vi "AlliGator Create Phasor Plot Additional Data String.vi"(4 "Intensity Weighted ? (F)":bool, 6 "Average Plot Data (F)":bool, 7 "Include Header String (F)":bool, 8 "error in (no error)":errorcluster, 9 "Calibrated Phasor Plot":T2, 10 "Raw Phasor Plot":T4={"Phasor Plot Name"="", "Raw Phasor Plot"=[], "Phasor Frequency"=0.0, "[Decay Metadata]"=[], "Raw Phasor Plot SDV"=[], "Phasor SDV Options"={"Compute Estimated SDV"=FALSE, "# Replicas"=100, "Use Estimated Average Phasor"=FALSE}, "[Calibration Phasor]"=[], "Intensity Array"=[]} {"[Decay Metadata]"."# Folds" min=1; "[Decay Metadata]"."ROI Descriptor"."Contours"."Type" items=["No Selection", "Point", "Line", "Rectangle", "Oval", "Polygon", "Freehand Region", "Annulus", "Unused2", "Unused3", "Broken Line", "Freehand Line", "Rotated Rectangle"]}, 11 "Phasor Plot Exported Data":T1) -> (0 "error out":errorcluster, 3 "Phasor Plot Additional Data String":string)   [LabVIEW 2021, in "AlliGator Phasor Graph.lvlib"]
doc: "Creates a string with all the user-requested phasor plot additional data."
uses:
  AlliGator Phasor Graph.lvlib
  AlliGator Raw Phasor Plot Data v5.ctl
  Phasor/Phasor (g, s).ctl
  AlliGator Decay Metadata v3.ctl
  Decay Analysis/Decay Preprocessing/AlliGator Decay Background Subtraction Info.ctl
  Decay Analysis/Decay Preprocessing/AlliGator Baseline Subtraction Method.ctl
  Graphs/XY Graph/XY Graph Plot Shift Parameters.ctl
  Graphs/XY Graph/XY Graph Plot Shift Method.ctl
  Decay Analysis/Decay Preprocessing/AlliGator Decay Extrapolation Parameters.ctl
  Phasor/Phasor Standard Deviation Options.ctl
  Phasor/Calibration Phasor (m, phi).ctl
  AlliGator Phasor Plot Additional Data List.ctl
  Graphs/XY Graph/XY Graph Plot Data.ctl
  AlliGator Phasor Plot Exported Data Selection.ctl
  d5eb63e0-648c-47d6-be91-64ae69301d4e.vi
  28782bb2-77f9-4fec-b09f-3ba0b8238253.vi
  Strings/Strings.lvlib
  Phasor/Phasor.lvlib
  Phasor Ratio/AlliGator Phasor Ratio.lvlib
  Time/Time.lvlib
  Utilities/Utilities.lvlib
  Math/Math.lvlib
  Decay Analysis/Decay Preprocessing/AlliGator Decay Preprocessing.lvlib
  Graphs/XY Graph/XY Graph Add-Ons.lvlib
panel:
  out "CPU (s)":dbl
  in  "Phasor Plot Exported Data List":T3
  # "see the AlliGator License on the block diagram (Ctrl+E or Window:Show Block Diagram)"
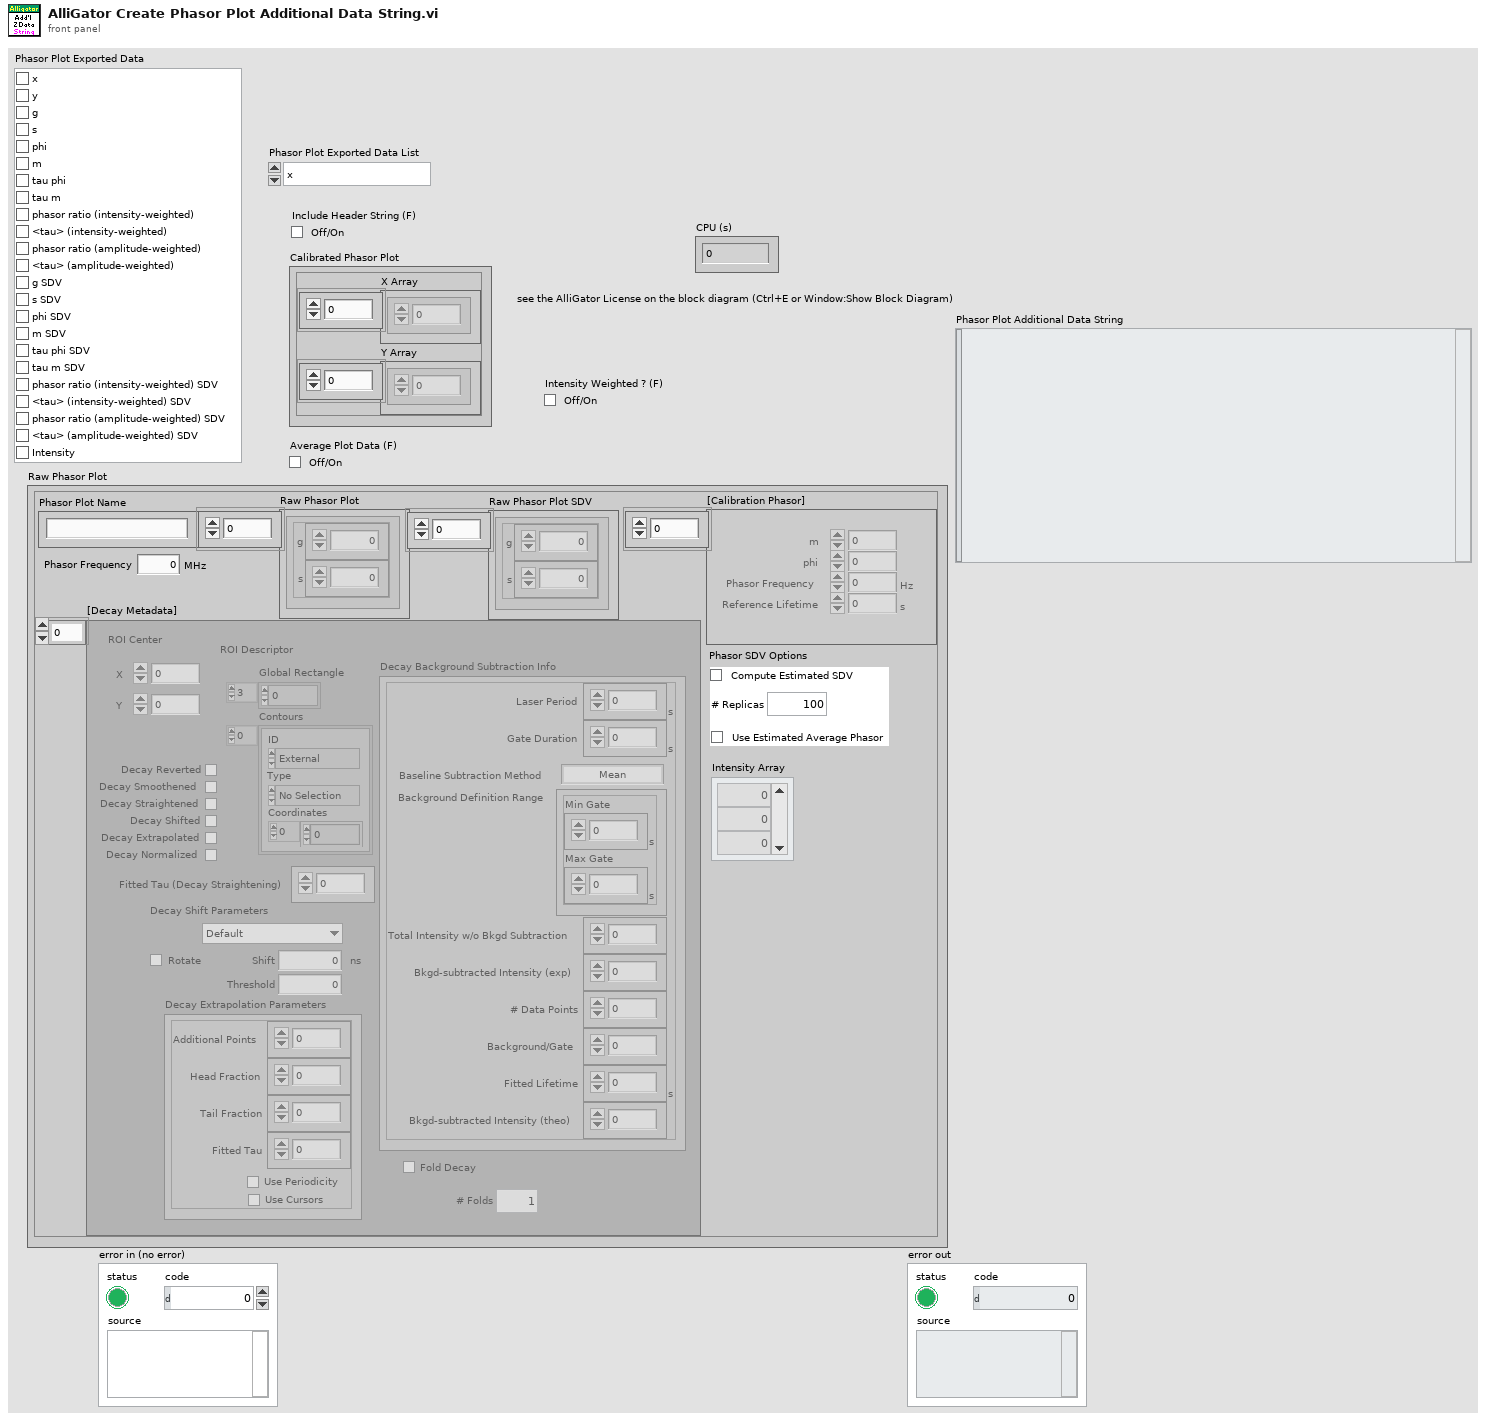
[diagram p1: front panel]
types:
  T1 = typedef "AlliGator Phasor Graph.lvlib/AlliGator Phasor Plot Exported Data Selection.ctl" = cluster{"x":bool, "y":bool, "g":bool, "s":bool, "phi":bool, "m":bool, "tau phi":bool, "tau m":bool, "phasor ratio (intensity-weighted)":bool, "<tau> (intensity-weighted)":bool, "phasor ratio (amplitude-weighted)":bool, "<tau> (amplitude-weighted)":bool, "g SDV":bool, "s SDV":bool, "phi SDV":bool, "m SDV":bool, "tau phi SDV":bool, "tau m SDV":bool, "phasor ratio (intensity-weighted) SDV":bool, "<tau> (intensity-weighted) SDV":bool, "phasor ratio (amplitude-weighted) SDV":bool, "<tau> (amplitude-weighted) SDV":bool, "Intensity":bool}
  T2 = typedef "XY Graph Add-Ons.lvlib/XY Graph Plot Data.ctl" = cluster{"X Array":dbl[], "Y Array":dbl[]}
  T3 = typedef "AlliGator Phasor Graph.lvlib/AlliGator Phasor Plot Additional Data List.ctl" = enum16{"x", "y", "g", "s", "phi", "m", "tau phi", "tau m", "phasor ratio (intensity-weighted)", "<tau> (intensity-weighted)", "phasor ratio (amplitude-weighted)", "<tau> (amplitude-weighted)", "g SDV", "s SDV", "phi SDV", "m SDV", "tau phi SDV", "tau m SDV", "phasor ratio (intensity-weighted) SDV", "<tau> (intensity-weighted) SDV", "phasor ratio (amplitude-weighted) SDV", "<tau> (amplitude-weighted) SDV", "Intensity"}
  T4 = typedef "AlliGator Phasor Graph.lvlib/AlliGator Raw Phasor Plot Data v5.ctl" = cluster{"Phasor Plot Name":string, "Raw Phasor Plot":T5[], "Phasor Frequency":dbl[unit], "[Decay Metadata]":T6[], "Raw Phasor Plot SDV":T5[], "Phasor SDV Options":T13, "[Calibration Phasor]":T14[], "Intensity Array":dbl[]}
  T5 = typedef "Phasor.lvlib/Phasor (g, s).ctl" = cluster{"g":dbl, "s":dbl}
  T6 = typedef "AlliGator Phasor Graph.lvlib/AlliGator Decay Metadata v3.ctl" = cluster{"ROI Descriptor":T7, "ROI Center":cluster{"X":i32, "Y":i32}, "Decay Background Subtraction Info":T8, "Decay Reverted":bool, "Decay Smoothened":bool, "Decay Straightened":bool, "Fitted Tau (Decay Straightening)":dbl, "Decay Shift Parameters":T10, "Decay Shifted":bool, "Decay Extrapolated":bool, "Decay Extrapolation Parameters":T12, "Decay Normalized":bool, "Fold Decay":bool, "# Folds":u32}
  T7 = typedef "ROI Descriptor" = cluster{"Global Rectangle":i32[], "Contours":cluster{"ID":enum32{"External", "Internal"}, "Type":u32, "Coordinates":i32[]}[]}
  T8 = typedef "AlliGator Decay Preprocessing.lvlib/AlliGator Decay Background Subtraction Info.ctl" = cluster{"Laser Period":dbl[unit], "Gate Duration":dbl[unit], "Baseline Subtraction Method":T9, "Background Definition Range":cluster{"Min Gate":dbl[unit], "Max Gate":dbl[unit]}, "Total Intensity w/o Bkgd Subtraction":dbl, "Bkgd-subtracted Intensity (exp)":dbl, "# Data Points":i32, "Background/Gate":dbl, "Fitted Lifetime":dbl[unit], "Bkgd-subtracted Intensity (theo)":dbl}
  T9 = typedef "AlliGator Decay Preprocessing.lvlib/AlliGator Baseline Subtraction Method.ctl" = enum16{"Mean", "Min", "Square Gated Single-Exponential", "File", "Constant"}
  T10 = typedef "XY Graph Add-Ons.lvlib/XY Graph Plot Shift Parameters.ctl" = cluster{"Type":T11, "Shift":dbl[unit], "Threshold":dbl, "Rotate":bool}
  T11 = typedef "XY Graph Add-Ons.lvlib/XY Graph Plot Shift Method.ctl" = enum16{"Default", "CFD", "Threshold", "Cross-Correlation"}
  T12 = typedef "AlliGator Decay Preprocessing.lvlib/AlliGator Decay Extrapolation Parameters.ctl" = cluster{"Additional Points":u32, "Head Fraction":dbl, "Fitted Tau":dbl, "Use Periodicity":bool, "Use Cursors":bool, "Tail Fraction":dbl}
  T13 = typedef "Phasor.lvlib/Phasor Standard Deviation Options.ctl" = cluster{"Compute Estimated SDV":bool, "# Replicas":u32, "Use Estimated Average Phasor":bool}
  T14 = typedef "Phasor.lvlib/Calibration Phasor (m, phi).ctl" = cluster{"m":dbl, "phi":dbl, "Phasor Frequency":dbl[unit], "Reference Lifetime":dbl[unit]}
  T15 = cluster{"Numeric Control":dbl, "Numeric Control":dbl}[]
  T16 = typedef "Phasor.lvlib/Phasor (m, phi).ctl" = cluster{"m":dbl, "phi":dbl}
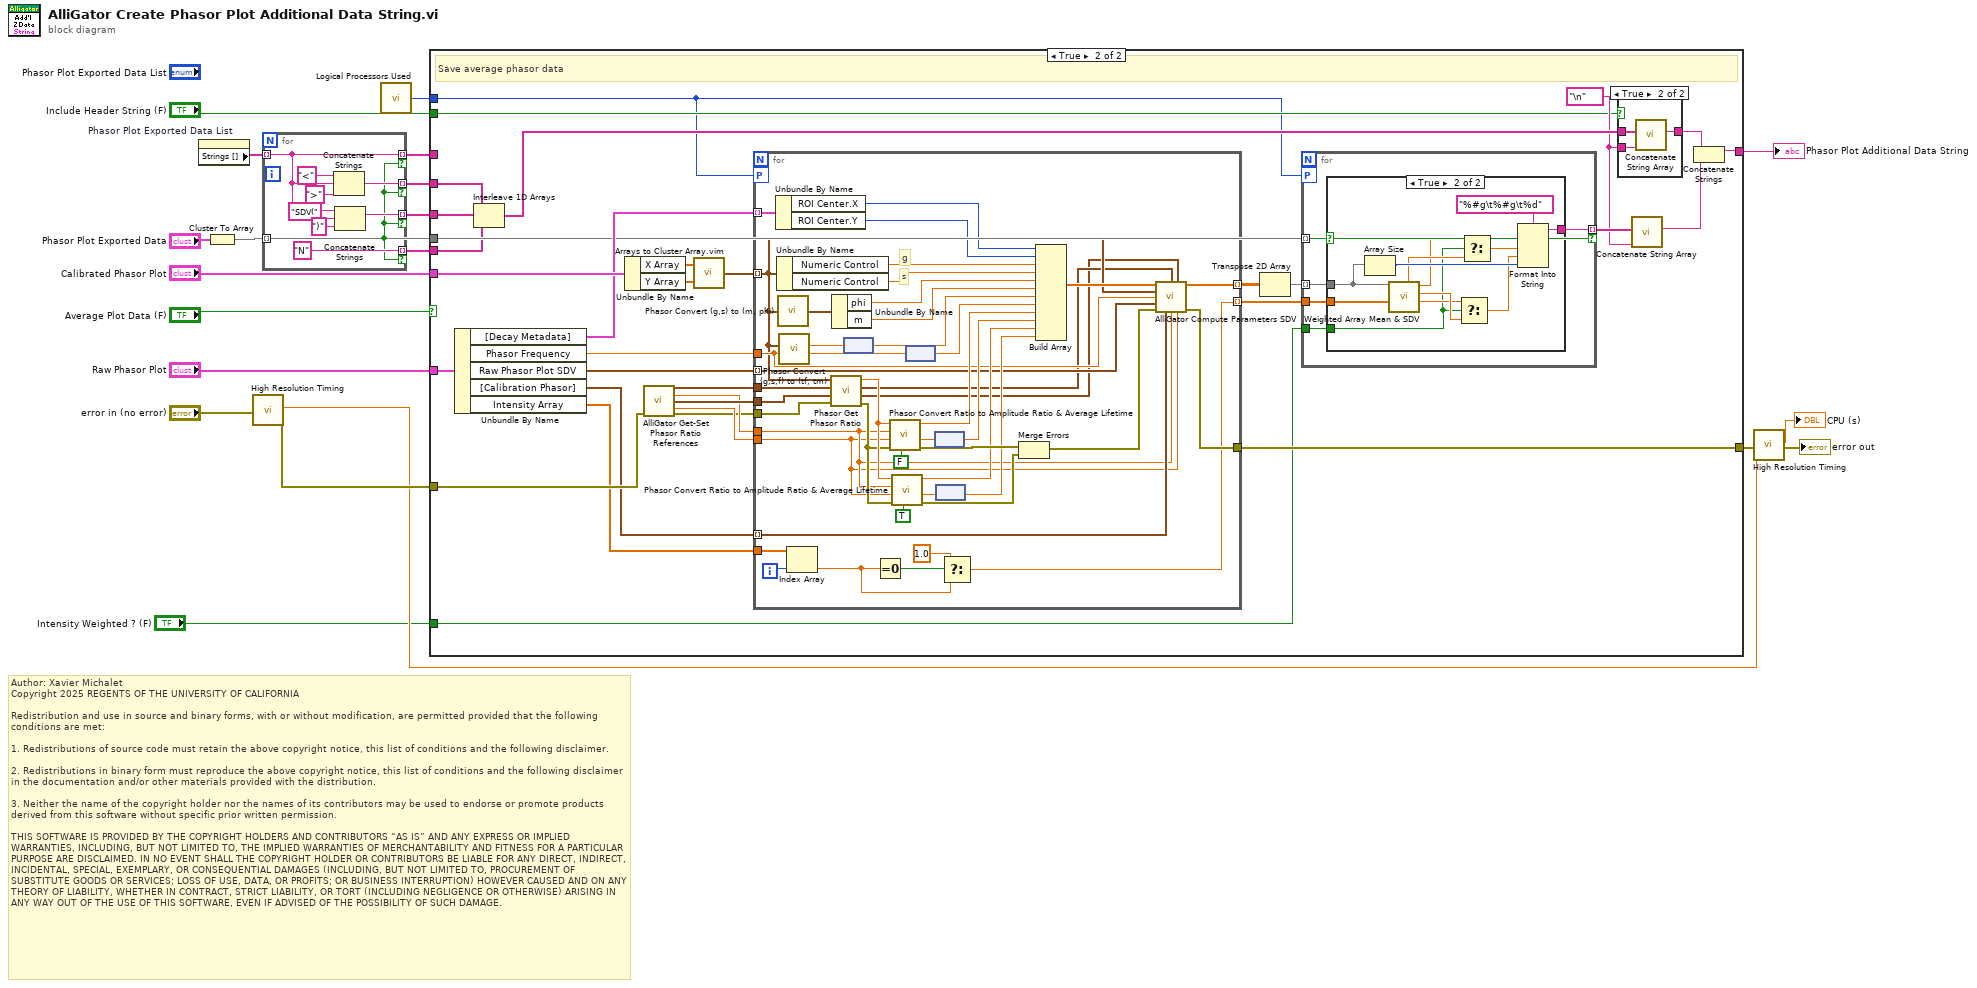
[diagram p0: block diagram]
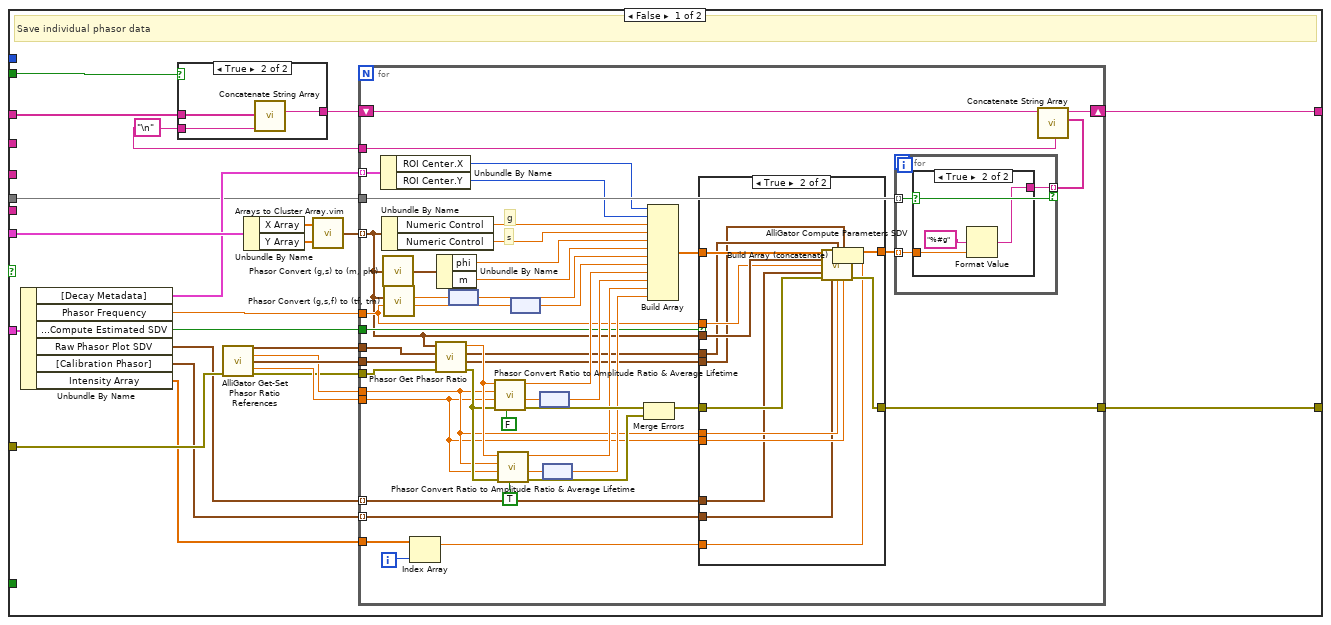
[diagram p2: hidden frame]
diagram:
  # "Author: Xavier Michalet\nCopyright 2025 REGENTS OF THE UNIVERSITY OF CALIFORNIA\n\nRedistribution and use in source and binary forms, with or without modification, are permitted provided that the following conditions are met:\n\n1. Redistributions of source code must retain the above copyright notice, this list of conditions and the following disclaimer.\n\n2. Redistributions in binary form must reproduce the above copyright notice, this list of conditions and the following disclaimer in the documentation and/or other materials provided with the distribution.\n\n3. Neither the name of the copyright holder nor the names of its contributors may be used to endorse or promote products derived from this software without specific prior written permission.\n\nTHIS SOFTWARE IS PROVIDED BY THE COPYRIGHT HOLDERS AND CONTRIBUTORS “AS IS” AND ANY EXPRESS OR IMPLIED WARRANTIES, INCLUDING, BUT NOT LIMITED TO, THE IMPLIED WARRANTIES OF MERCHANTABILITY AND FITNESS FOR A PARTICULAR PURPOSE ARE DISCLAIMED. IN NO EVENT SHALL THE COPYRIGHT HOLDER OR CONTRIBUTORS BE LIABLE FOR ANY DIRECT, INDIRECT, INCIDENTAL, SPECIAL, EXEMPLARY, OR CONSEQUENTIAL DAMAGES (INCLUDING, BUT NOT LIMITED TO, PROCUREMENT OF SUBSTITUTE GOODS OR SERVICES; LOSS OF USE, DATA, OR PROFITS; OR BUSINESS INTERRUPTION) HOWEVER CAUSED AND ON ANY THEORY OF LIABILITY, WHETHER IN CONTRACT, STRICT LIABILITY, OR TORT (INCLUDING NEGLIGENCE OR OTHERWISE) ARISING IN ANY WAY OUT OF THE USE OF THIS SOFTWARE, EVEN IF ADVISED OF THE POSSIBILITY OF SUCH DAMAGE."
  n1 = property on="Phasor Plot Exported Data List" class="Enum (strict)"() -> ("Strings []"=w20:string[])  [unwired: 2 in, 2 out]
  n2 = Cluster To Array(cluster="Phasor Plot Exported Data") -> (array=w14:bool[])
  n3 = call "High Resolution Timing.vi"("Error In"="error in (no error)") -> ("elapsed (relative) seconds"=w9:dbl, "Error Out"=w11:errorcluster)  [unwired: 16 in, 1 out]
  n4 = for {
    tunnel: w14 -> [w21] mode=indexing
    tunnel: w20 -> [w24] mode=indexing
    tunnel: [w24] -> w17 mode=indexing if=w21
    tunnel: [w27] -> w6 mode=indexing if=w21
    tunnel: [w26] -> w5 mode=indexing if=w21
    tunnel: ["N" ("string")] -> w3 mode=indexing if=w21
    n5 = Concatenate Strings("<" ("string"), w24, ">" ("string")) -> (w27:string)
    n6 = Concatenate Strings("SDV(" ("string"), w24, ")" ("string")) -> (w26:string)
  }
  n7 = call "Logical Processors Used.vi"() -> ("# Logical Processor Used"=w2:i32)  [unwired: 6 in]
  n8 = case shown="True" "Average Plot Data (F)" {
    tunnel: "Raw Phasor Plot" -> [w48 w157]
    tunnel: "Calibrated Phasor Plot" -> [w53 w161]
    tunnel: w17 -> [w49 _]
    tunnel: w11 -> [w41 w150]
    tunnel: w14 -> [w36 w142]
    tunnel: [w39 w137] -> w13
    tunnel: [w38 w149] -> w12
    tunnel: w6 -> [_ w147]
    tunnel: w5 -> [_ w146]
    tunnel: "Include Header String (F)" -> [w35 w136]
    tunnel: w3 -> [_ w135]
    tunnel: w2 -> [_ w134]
    tunnel: "Intensity Weighted ? (F)" -> [_ w129]
    frame False {
      w34 = "\n"
      # "Save individual phasor data"
      n9 = Unbundle By Name(w48) -> ("[Decay Metadata]"=w37:T6[], "Phasor Frequency"=w47:dbl[unit], "Phasor SDV Options.Compute Estimated SDV"=w31:bool, "Raw Phasor Plot SDV"=w33:T5[], "[Calibration Phasor]"=w32:T14[], "Intensity Array"=w30:dbl[])
      n10 = case shown="True" w35 {
        tunnel: w49 -> [_ w128]
        tunnel: [_ w127] -> w40
        tunnel: w34 -> [_ w126]
        frame False {
        }
        frame True {
          n11 = call "Concatenate String Array.vi"("Suffix (\"\")"=w126, "String Array"=w128) -> ("Formatted String"=w127:string)  [unwired: 9 in]
        }
      }
      n12 = call "AlliGator Get-Set Phasor Ratio References.vi"("error in (no error)"=w41) -> ("Reference Phasor 1"=w46:T5, "Reference Lifetime 1"=w44:dbl[unit], "Reference Phasor 2"=w45:T5, "Reference Lifetime 2"=w43:dbl[unit], "error out"=w42:errorcluster)  [unwired: 7 in, 3 out]
      n13 = Unbundle By Name(w53) -> ("X Array"=w52:dbl[], "Y Array"=w51:dbl[])
      n14 = call "Arrays to Cluster Array.vim"("Array 1"=w52, "Array 2"=w51) -> ("Cluster Array"=w50:T15)  [unwired: 6 in]
      n15 = for {
        tunnel: w50 -> [w61] mode=indexing
        tunnel: w47 -> [w62]
        tunnel: w46 -> [w60]
        tunnel: w45 -> [w59]
        tunnel: w44 -> [w58]
        tunnel: w43 -> [w57]
        tunnel: w42 -> [w96]
        shift-right: [w83] -> w39
        shift-left: w40 -> [w84]
        tunnel: w36 -> [w86]
        tunnel: w34 -> [w82]
        tunnel: [w64] -> w38
        tunnel: w37 -> [w80] mode=indexing
        tunnel: w33 -> [w66] mode=indexing
        tunnel: w32 -> [w63] mode=indexing
        tunnel: w31 -> [w69]
        tunnel: w30 -> [w56]
        i -> [w55]
        # "s"
        # "g"
        n16 = Unbundle By Name(w80) -> ("ROI Center.X"=w79:i32, "ROI Center.Y"=w78:i32)
        n17 = Unbundle By Name(w61) -> ("Numeric Control"=w94:dbl, "Numeric Control"=w93:dbl)
        n18 = call "Phasor Convert (g,s) to (m, phi).vi"("Phasor (g, s)"=w61) -> ("Phasor (m, phi)"=w99:T16)  [unwired: 8 in]
        n19 = call "Phasor Convert (g,s,f) to (tf, tm).vi"("Phasor Harmonic Frequency"=w62, "Phasor (g, s)"=w61) -> ("Modulus Lifetime"=w97:dbl[unit], "Phase Lifetime"=w98:dbl[unit])  [unwired: 7 in, 1 out]
        n20 = Index Array(array=w56, index=w55) -> (element=w54:dbl)
        n21 = call "Phasor Get Phasor Ratio.vi"("Error In"=w96, "Reference Phasor 2"=w59, "Reference Phasor 1"=w60, "Phasor"=w61) -> ("Error Out"=w73:errorcluster, "Phasor Ratio (f1)"=w74:dbl)  [unwired: 5 in, 1 out]
        n22 = Unbundle By Name(w99) -> ("phi"=w92:dbl, "m"=w91:dbl)
        n23 = node(w98) -> (w90:dbl)
        n24 = call "Phasor Convert Ratio to Amplitude Ratio & Average Lifetime.vi"("Compute Amplitude Ratio"=FALSE, "error in (no error)"=w73, "Reference Lifetime 2"=w57, "Reference Lifetime 1"=w58, "Phasor Ratio (f1)"=w74) -> ("error out"=w81:errorcluster, "Average Lifetime"=w95:dbl[unit], "Phasor/Amplitude Ratio"=w88:dbl)  [unwired: 2 in, 2 out]
        n25 = call "Phasor Convert Ratio to Amplitude Ratio & Average Lifetime.vi"("Compute Amplitude Ratio"=TRUE, "error in (no error)"=w73, "Reference Lifetime 2"=w57, "Reference Lifetime 1"=w58, "Phasor Ratio (f1)"=w74) -> ("error out"=w70:errorcluster, "Average Lifetime"=w76:dbl[unit], "Phasor/Amplitude Ratio"=w72:dbl)  [unwired: 2 in, 2 out]
        n26 = node(w97) -> (w89:dbl)
        n27 = node(w95) -> (w87:dbl)
        n28 = node(w76) -> (w71:dbl)
        n29 = Merge Errors(w81, w70) -> (w65:errorcluster)
        n30 = Build Array(w79, w78, w94, w93, w92, w91, w90, w89, w88, w87, w72, w71) -> (w68:dbl[])
        n31 = case shown="True" w69 {
          tunnel: w68 -> [w105 w119]
          tunnel: [w104 w107] -> w67
          tunnel: w66 -> [_ w113]
          tunnel: w65 -> [w100 w116]
          tunnel: [w100 w117] -> w64
          tunnel: w63 -> [_ w108]
          tunnel: w62 -> [_ w111]
          tunnel: w61 -> [_ w112]
          tunnel: w60 -> [_ w110]
          tunnel: w59 -> [_ w109]
          tunnel: w58 -> [_ w115]
          tunnel: w57 -> [_ w114]
          tunnel: w54 -> [_ w106]
          frame False {
            # "no SDV estimated"
            n32 = Initialize Array(0.0 ("Numeric Control"), 10 ("dimension size")) -> (w103:dbl[])
            n33 = Build Array (concatenate)(w105, w103) -> (w104:dbl[])
          }
          frame True {
            n34 = call "AlliGator Compute Parameters SDV.vi"("Parameters in"=w119, "Reference Phasor 1"=w110, "Reference Phasor 2"=w109, "Phasor"=w112, "Phasor Frequency"=w111, "Raw Phasor SDV"=w113, "error in (no error)"=w116, "Calibration Phasor"=w108, "Reference Lifetime 1"=w115, "Reference Lifetime 2"=w114) -> ("Parameters out"=w118:dbl[], "error out"=w117:errorcluster)  [unwired: 4 in]
            n35 = Build Array (concatenate)(w118, w106) -> (w107:dbl[])
          }
        }
        n36 = for {
          tunnel: w86 -> [w120] mode=indexing
          tunnel: w67 -> [w122] mode=indexing
          tunnel: [w121] -> w85 mode=indexing if=w120
          n37 = case shown="True" w120 {
            tunnel: w122 -> [_ w125]
            tunnel: [_ w123] -> w121
            frame False {
            }
            frame True {
              n38 = Format Value(format string="%#g", value (0)=w125) -> (output string=w123:string)  [unwired: 1 in]
            }
          }
        }
        n39 = call "Concatenate String Array.vi"("Suffix (\"\")"=w82, "String Array"=w85, "Prefix (\"\")"=w84) -> ("Formatted String"=w83:string)  [unwired: 8 in]
      }
    }
    frame True {
      w140 = "\n"
      # "Save average phasor data"
      n40 = Unbundle By Name(w157) -> ("[Decay Metadata]"=w148:T6[], "Phasor Frequency"=w156:dbl[unit], "Raw Phasor Plot SDV"=w133:T5[], "[Calibration Phasor]"=w132:T14[], "Intensity Array"=w131:dbl[])
      n41 = Interleave 1D Arrays(w147, w146, w135) -> (w145:string[])
      n42 = Unbundle By Name(w161) -> ("X Array"=w160:dbl[], "Y Array"=w159:dbl[])
      n43 = call "AlliGator Get-Set Phasor Ratio References.vi"("error in (no error)"=w150) -> ("Reference Phasor 1"=w155:T5, "Reference Lifetime 1"=w153:dbl[unit], "Reference Phasor 2"=w154:T5, "Reference Lifetime 2"=w152:dbl[unit], "error out"=w151:errorcluster)  [unwired: 7 in, 3 out]
      n44 = call "Arrays to Cluster Array.vim"("Array 1"=w160, "Array 2"=w159) -> ("Cluster Array"=w158:T15)  [unwired: 6 in]
      n45 = for {
        tunnel: w158 -> [w194] mode=indexing
        tunnel: w156 -> [w195]
        tunnel: w155 -> [w192]
        tunnel: w154 -> [w191]
        tunnel: w153 -> [w189]
        tunnel: w152 -> [w188]
        tunnel: w151 -> [w221]
        tunnel: [w196] -> w149
        tunnel: w148 -> [w210] mode=indexing
        tunnel: [w198] -> w144 mode=indexing
        workers-P: w134 -> [_]
        tunnel: w133 -> [w193] mode=indexing
        tunnel: w132 -> [w190] mode=indexing
        tunnel: w131 -> [w187]
        tunnel: [w182] -> w130 mode=indexing
        i -> [w186]
        # "s"
        # "g"
        n46 = Unbundle By Name(w210) -> ("ROI Center.X"=w209:i32, "ROI Center.Y"=w208:i32)
        n47 = Unbundle By Name(w194) -> ("Numeric Control"=w219:dbl, "Numeric Control"=w218:dbl)
        n48 = call "Phasor Convert (g,s) to (m, phi).vi"("Phasor (g, s)"=w194) -> ("Phasor (m, phi)"=w224:T16)  [unwired: 8 in]
        n49 = call "Phasor Convert (g,s,f) to (tf, tm).vi"("Phasor Harmonic Frequency"=w195, "Phasor (g, s)"=w194) -> ("Modulus Lifetime"=w222:dbl[unit], "Phase Lifetime"=w223:dbl[unit])  [unwired: 7 in, 1 out]
        n50 = Index Array(array=w187, index=w186) -> (element=w183:dbl)
        n51 = call "Phasor Get Phasor Ratio.vi"("Error In"=w221, "Reference Phasor 2"=w191, "Reference Phasor 1"=w192, "Phasor"=w194) -> ("Error Out"=w201:errorcluster, "Phasor Ratio (f1)"=w206:dbl)  [unwired: 5 in, 1 out]
        n52 = Unbundle By Name(w224) -> ("phi"=w217:dbl, "m"=w216:dbl)
        n53 = node(w223) -> (w215:dbl)
        n54 = Equal To 0?(x=w183) -> (x = 0?=w185:bool)
        n55 = call "Phasor Convert Ratio to Amplitude Ratio & Average Lifetime.vi"("Compute Amplitude Ratio"=FALSE, "error in (no error)"=w201, "Reference Lifetime 2"=w188, "Reference Lifetime 1"=w189, "Phasor Ratio (f1)"=w206) -> ("error out"=w211:errorcluster, "Average Lifetime"=w220:dbl[unit], "Phasor/Amplitude Ratio"=w213:dbl)  [unwired: 2 in, 2 out]
        n56 = call "Phasor Convert Ratio to Amplitude Ratio & Average Lifetime.vi"("Compute Amplitude Ratio"=TRUE, "error in (no error)"=w201, "Reference Lifetime 2"=w188, "Reference Lifetime 1"=w189, "Phasor Ratio (f1)"=w206) -> ("error out"=w200:errorcluster, "Average Lifetime"=w204:dbl[unit], "Phasor/Amplitude Ratio"=w203:dbl)  [unwired: 2 in, 2 out]
        n57 = node(w222) -> (w214:dbl)
        n58 = node(w220) -> (w212:dbl)
        n59 = node(w204) -> (w202:dbl)
        n60 = Select(t=1.0 ("element"), s=w185, f=w183) -> (s? t:f=w182:dbl)
        n61 = Merge Errors(w211, w200) -> (w197:errorcluster)
        n62 = Build Array(w209, w208, w219, w218, w217, w216, w215, w214, w213, w212, w203, w202) -> (w199:dbl[])
        n63 = call "AlliGator Compute Parameters SDV.vi"("Parameters in"=w199, "Reference Phasor 1"=w192, "Reference Phasor 2"=w191, "Phasor"=w194, "Phasor Frequency"=w195, "Raw Phasor SDV"=w193, "error in (no error)"=w197, "Calibration Phasor"=w190, "Reference Lifetime 1"=w189, "Reference Lifetime 2"=w188) -> ("Parameters out"=w198:dbl[], "error out"=w196:errorcluster)  [unwired: 4 in]
      }
      n64 = Transpose 2D Array(2D array=w144) -> (transposed array=w143:dbl[][])
      n65 = for {
        tunnel: w143 -> [w169] mode=indexing
        tunnel: w142 -> [w167] mode=indexing
        tunnel: [w168] -> w141 mode=indexing if=w167
        workers-P: w134 -> [_]
        tunnel: w130 -> [w166]
        tunnel: w129 -> [w165]
        n66 = case shown="True" w167 {
          tunnel: w169 -> [_ w178]
          tunnel: [_ w180] -> w168
          tunnel: w166 -> [_ w179]
          tunnel: w165 -> [_ w172]
          frame False {
          }
          frame True {
            n67 = Array Size(array=w178) -> (size(s)=w177:i32)
            n68 = call "Weighted Array Mean & SDV.vi"("Weight Array"=w179, "Array"=w178) -> ("SDV (weighted)"=w175:dbl, "SDV (classic)"=w176:dbl, "Average Value (weighted)"=w171:dbl, "Average Value (classic)"=w173:dbl)  [unwired: 4 in, 2 out]
            n69 = Select(t=w175, s=w172, f=w176) -> (s? t:f=w174:dbl)
            n70 = Select(t=w171, s=w172, f=w173) -> (s? t:f=w170:dbl)
            n71 = Format Into String(format string="%#g\t%#g\t%d", w170, w174, w177) -> (resulting string=w180:string)  [unwired: 2 in, 1 out]
          }
        }
      }
      n72 = case shown="True" w136 {
        tunnel: w145 -> [_ w164]
        tunnel: w140 -> [_ w163]
        tunnel: [_ w162] -> w139
        frame False {
        }
        frame True {
          n73 = call "Concatenate String Array.vi"("Suffix (\"\")"=w163, "String Array"=w164) -> ("Formatted String"=w162:string)  [unwired: 9 in]
        }
      }
      n74 = call "Concatenate String Array.vi"("Suffix (\"\")"=w140, "String Array"=w141) -> ("Formatted String"=w138:string)  [unwired: 9 in]
      n75 = Concatenate Strings(w139, w138) -> (w137:string)
    }
  }
  "Phasor Plot Additional Data String" <- w13
  n76 = call "High Resolution Timing.vi"("relative seconds (NaN)"=w9, "Error In"=w12) -> ("elapsed (relative) seconds"=→"CPU (s)":dbl, "Error Out"=→"error out":errorcluster)  [unwired: 15 in, 1 out]
